vi "Get List of Files for Hash.vi"(8 "error in":errorcluster, 11 "Peer Review in":refnum<class "Peer Review.lvclass">) -> (0 "error out":errorcluster, 3 "Peer Review out":refnum<class "Peer Review.lvclass">)   [LabVIEW 2020, in "Peer Review.lvclass"]
uses:
  Peer Review.lvclass
  Peer Review.lvclass/Peer Review.ctl
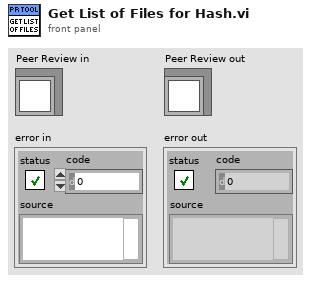
[diagram p1: front panel]
types:
  T1 = typedef "Peer Review.lvclass/Commit Info.ctl" = cluster{"Commit ID":i32, "Hash":string, "Merge Commit?":bool, "Merge Hash":string, "Author":string, "Time Stamp":timestamp, "Description":string, "File Count":i32, "File List":string[]}
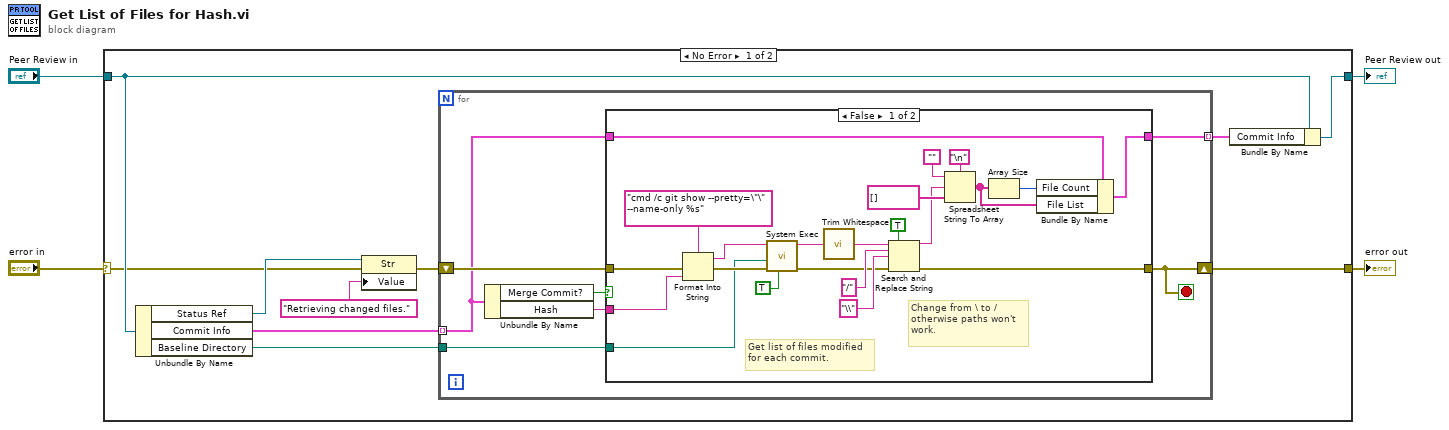
[diagram p0: block diagram]
diagram:
  n1 = case shown="No Error" "error in" {
    selector: "error in" -> [w6 w47]
    tunnel: [w14 w47] -> w3
    tunnel: [w10 w46] -> w1
    tunnel: "Peer Review in" -> [w9 w46]
    frame No Error {
      n2 = Unbundle By Name(w9) -> ("Status Ref"=w7:refnum<vi>, "Commit Info"=w12:T1[], "Baseline Directory"=w13:path)
      n3 = property on="Property Node" class="Str"(reference=w7, error in=w6, "Value"="Retrieving changed files.") -> (error out=w5:errorcluster)  [unwired: 1 out]
      n4 = for {
        shift-right: [w15] -> w14
        shift-left: w5 -> [w21]
        tunnel: w13 -> [w20]
        tunnel: w12 -> [w17] mode=indexing
        tunnel: [w16] -> w11 mode=indexing
        stop <- w15 stop-if-true
        n5 = Unbundle By Name(w17) -> ("Merge Commit?"=w18:bool, "Hash"=w19:string)
        n6 = case shown="False" w18 {
          tunnel: [w24 w44] -> w15
          tunnel: w21 -> [w42 w44]
          tunnel: w20 -> [w37 _]
          tunnel: w19 -> [w33 _]
          tunnel: w17 -> [w32 w45]
          tunnel: [w30 w45] -> w16
          frame False {
            # "Change from \\ to /\notherwise paths won't\nwork."
            # "Get list of files modified\nfor each commit."
            n7 = Format Into String(format string="cmd /c git show --pretty=\"\" --name-only %s" ("command line"), error in=w42, w33) -> (resulting string=w39:string, error out=w41:errorcluster)  [unwired: 1 in]
            n8 = call <vilib>:"System Exec.vi"("run minimized? (F)"=TRUE, "error in (no error)"=w41, "working directory"=w37, "command line"=w39) -> ("error out"=w25:errorcluster, "standard output"=w38:string)  [unwired: 4 in, 2 out]
            n9 = call <vilib>:"Trim Whitespace.vi"("string"=w38) -> ("trimmed string"=w23:string)  [unwired: 1 in]
            n10 = Search and Replace String(replace all?=TRUE ("replace all? (F)"), input string=w23, search string="/", replace string="\\" ("search string"), error in=w25) -> (result string=w22:string, error out=w24:errorcluster)  [unwired: 3 in, 2 out]
            n11 = Spreadsheet String To Array(delimiter (Tab)="\n" ("Line Feed Constant"), format string="" ("Empty String Constant"), spreadsheet string=w22, array type (2D Dbl)=string[] []) -> (array=w29:string[])
            n12 = Array Size(array=w29) -> (size(s)=w31:i32)
            n13 = Bundle By Name(cluster=w32, "File Count"=w31, "File List"=w29) -> (w30:T1)
          }
          frame True {
            # "Disregard if a merge commit."
          }
        }
      }
      n14 = Bundle By Name(cluster=w9, "Commit Info"=w11) -> (w10:refnum<class "Peer Review.lvclass">)
    }
    frame Error {
    }
  }
  "error out" <- w3
  "Peer Review out" <- w1
